vi "Create.vi"(7 "Group":string="Default", 8 "error in (no error)":errorcluster, 10 "Tag":string, 11 "Blackboard":refnum<class "Blackboard.lvclass">) -> (0 "error out":errorcluster, 2 "Blackboard_Boolean.lvclass":refnum<class "Blackboard_Boolean.lvclass">, 3 "Blackboard Out":refnum<class "Blackboard.lvclass">)   [LabVIEW 2021, in "Blackboard_Boolean.lvclass"]
uses:
  Blackboard_Boolean.lvclass
  C:/Program Files (x86)/National Instruments/LabVIEW 2021/vi.lib/TSA/Abstract Data Classes/Abs_Types/Type/Abs_Type.lvclass
  Blackboard.lvclass
  Blackboard_Boolean.lvclass/Blackboard_Boolean.ctl
  <vilib>/TSA/Abstract Data Classes/Abs_Types/Type/Abs_Type.lvclass/Abs_Type.ctl
  Properties/Write Blackboard.vi
  Properties/Write Group.vi
  Properties/Write Write.vi
  <vilib>/TSA/Abstract Data Classes/Abs_Types/Type/Abs_Type.lvclass
  C:/Program Files (x86)/National Instruments/LabVIEW 2021/vi.lib/TSA/Abstract Data Classes/Abs_Types/Boolean/Abs_Boolean.lvclass
  C:/Program Files (x86)/National Instruments/LabVIEW 2021/vi.lib/TSA/Abstract Data Classes/Abs_Types/Value/Abs_Value.lvclass
  C:/Users/Tim/Documents/GitHub/LV_Behaviour_Tree/Source/Blackboard/Support/Bool/Blackboard_Boolean.lvclass
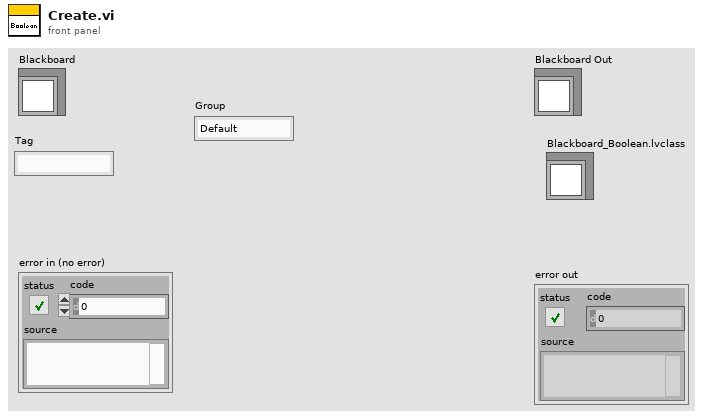
[diagram p1: front panel]
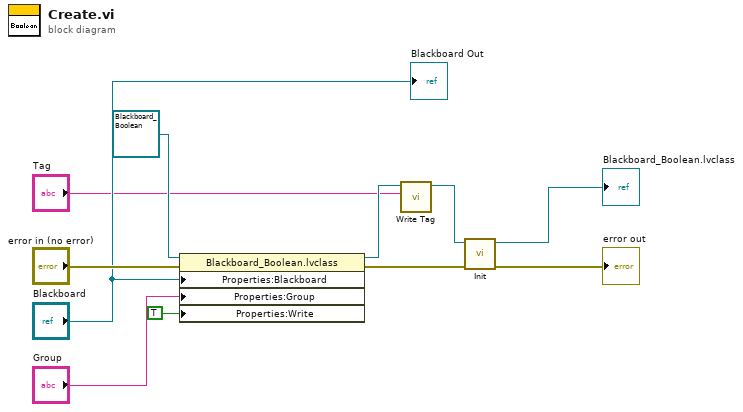
[diagram p0: block diagram]
diagram:
  n1 = property class="Blackboard_Boolean.lvclass"(reference=refnum<class "Blackboard_Boolean.lvclass"> refnum ("Blackboard_Boolean.lvclass"), error in="error in (no error)", "Properties:Blackboard"="Blackboard", "Properties:Group"="Group", "Properties:Write"=TRUE ("Write")) -> (reference out=w6:refnum<class "Blackboard_Boolean.lvclass">, error out=w3:errorcluster)
  n2 = call <vilib>:"Write Tag.vi"("Tag"="Tag", "Abs_Type in"=w6) -> ("Abs_Type out"=w5:refnum<class "Blackboard_Boolean.lvclass">)  [unwired: 9 in]
  n3 = call-dynamic "Init.vi"("error in (no error)"=w3, "Data in"=w5) -> ("error out"=→"error out":errorcluster, "Data out"=→"Blackboard_Boolean.lvclass":refnum<class "Blackboard_Boolean.lvclass">)  [unwired: 8 in]
  "Blackboard Out" <- "Blackboard"
